vi "Hardware in the Loop - Download Data (Multiplexed - Signed 32 Bit).vi"(8 "error in":errorcluster, 9 "Number of Samples":u32, 10 "Number of Channels":u32, 11 "Address":string) -> (0 "error out":errorcluster, 1 "Data Received":bool, 2 "Data":i32[][](array[numeric]))   [LabVIEW 2017, in "Communications Library.lvlib"]
doc: "Downloads multiplexed data from the DTACQ device, in 32 bit integer format, and reformats the data into a 2D array."
uses:
  Communications Library.lvlib
  Typedefs/Functional Global Variable Action--Enum.ctl
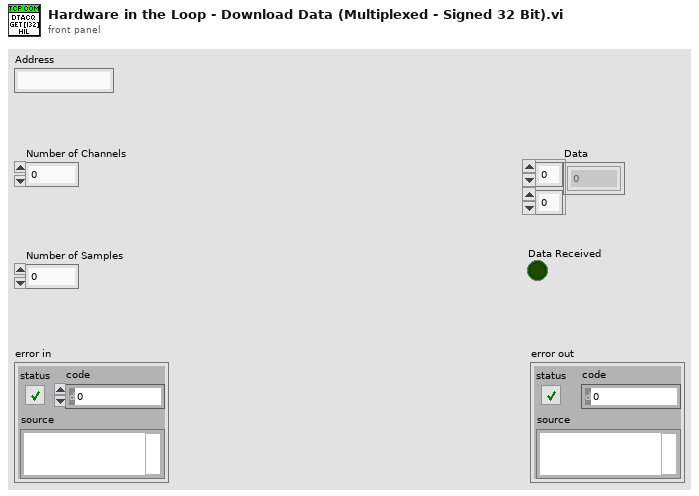
[diagram p1: front panel]
types:
  T1 = typedef "Communications Library.lvlib/Functional Global Variable Action--Enum.ctl" = enum16{"Initialise", "Write Module Config", "Write Carrier Config", "Read"}
  T2 = typedef "Communications Library.lvlib/DTACQ Module Carrier Configuration--Cluster.ctl" = cluster{"Name":string, "IP":string, "Control Port":i32, "Timeout (ms)":i32, "Continuous Capture Port (Multiplexed)":i32, "Start HIL Shot Port":i32, "AWG Upload Port (Multiplexed)":i32, "Download Captured Data Port (Multiplexed)":i32, "Module Slots":i32, "Module Configurations":T3[]}
  T3 = typedef "Communications Library.lvlib/DTACQ Module Configuration--Cluster.ctl" = cluster{"Name":string, "Position":string, "Module Type":T4, "Control Port":i32, "Timeout (ms)":i32, "Channels":i32}
  T4 = typedef "Communications Library.lvlib/DTACQ Device Type--Enum.ctl" = enum16{"Carrier", "Analog In Module", "Analog Out Module", "Generic Module"}
  T5 = typedef "Communications Library.lvlib/DTACQ Connection Data--Cluster.ctl" = cluster{"Description":string, "Address":string, "Port":u16, "timeout (ms)":i32, "Termination Character":string, "TCP Connection Reference":refnum<k5>, "Open Connection":bool}
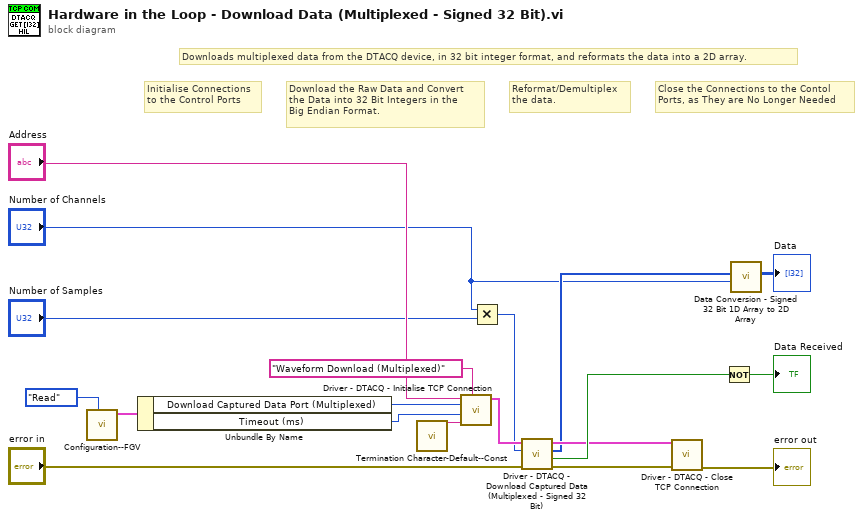
[diagram p0: block diagram]
diagram:
  # "Downloads multiplexed data from the DTACQ device, in 32 bit integer format, and reformats the data into a 2D array."
  # "Close the Connections to the Contol\nPorts, as They are No Longer Needed"
  # "Reformat/Demultiplex\nthe data."
  # "Download the Raw Data and Convert\nthe Data into 32 Bit Integers in the\nBig Endian Format."
  # "Initialise Connections\nto the Control Ports"
  n1 = call "Configuration--FGV.vi"("Functional Global Action"=Functional_Global_Variable_Action--Enum."Read") -> ("Carrier Configuration Out"=w12:T2)  [unwired: 9 in, 1 out]
  n2 = Unbundle By Name(w12) -> ("Download Captured Data Port (Multiplexed)"=w11:i32, "Timeout (ms)"=w10:i32)
  n3 = call "Termination Character-Default--Const.vi"() -> ("Termination Character"=w14:string)  [unwired: 11 in]
  n4 = call "Driver - DTACQ - Initialise TCP Connection.vi"("Description"="Waveform Download (Multiplexed)", "Termination Character"=w14, "timeout (ms)"=w10, "Port"=w11, "Address"="Address") -> ("DTACQ Connection Data Out"=w7:T5)  [unwired: 6 in]
  n5 = Multiply(x="Number of Channels", y="Number of Samples") -> (x*y=w6:u32)
  n6 = call "Driver - DTACQ - Download Captured Data (Multiplexed - Signed 32 Bit).vi"("error in"="error in", "Samples"=w6, "DTACQ Connection Data In"=w7) -> ("error out"=w9:errorcluster, "Timed Out"=w5:bool, "(Signed) 32 Bit Array"=w3:i32[], "DTACQ Connection Data Out"=w4:T5)  [unwired: 5 in]
  n7 = call "Driver - DTACQ - Close TCP Connection.vi"("error in"=w9, "DTACQ Connection Data In"=w4) -> ("error out"=→"error out":errorcluster)  [unwired: 8 in, 1 out]
  n8 = Not(x=w5) -> (.not. x?=→"Data Received":bool)
  n9 = call "Data Conversion - Signed 32 Bit 1D Array to 2D Array.vi"("Channels"="Number of Channels", "1D Data (Multiplexed)"=w3) -> ("2D Data (De-Multiplexed)"=→"Data":i32[][])  [unwired: 9 in]
